vi "TestABlock.vi"   [LabVIEW 2015]
doc: "This block is for testing other ESP301 Blocks. Basically it became too annoying to haveto add the connect and disconnect blocks to everything especially if something is not supposed to be a standalone program."
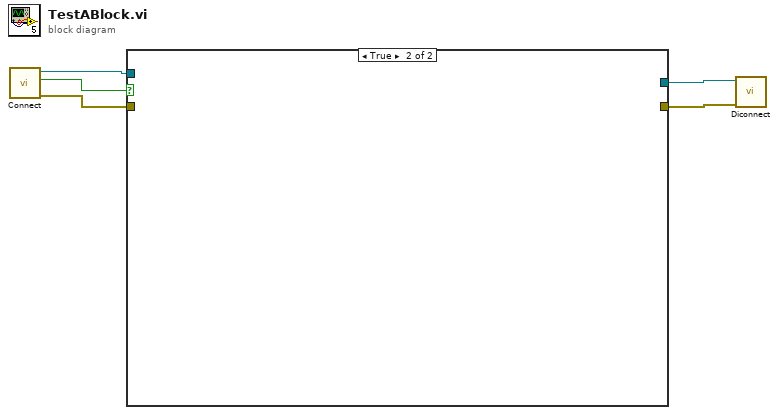
[diagram p0: block diagram]
diagram:
  n1 = call "Connect.vi"() -> ("error out"=w3:errorcluster, "Connected"=w5:bool, "VISA resource name out"=w4:refnum<visa-resource-name>)  [unwired: 5 in]
  n2 = case shown="True" w5 {
    tunnel: w4 -> [w7 _]
    tunnel: w3 -> [w6 _]
    tunnel: [w7 _] -> w2
    tunnel: [w6 _] -> w1
    frame False {
    }
    frame True {
    }
  }
  n3 = call "Diconnect.vi"("error in (no error)"=w1, "VISA resource name"=w2) -> ()  [unwired: 6 in]
